vi "initBufferRead.vi"(8 "error in (no error)":errorcluster, 10 "bufferSize":u32=50000, 11 "Electrometer in":refnum<class "Electrometer.lvclass">) -> (0 "error out":errorcluster, 3 "Electrometer out":refnum<class "Electrometer.lvclass">)   [LabVIEW 2016, in "Electrometer.lvclass"]
uses:
  Electrometer.lvclass
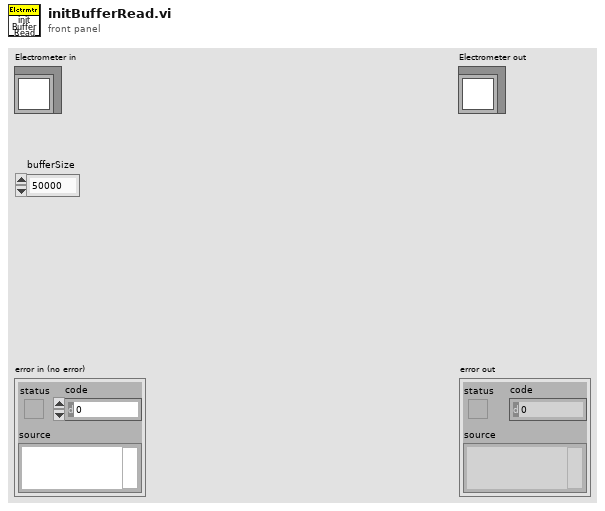
[diagram p1: front panel]
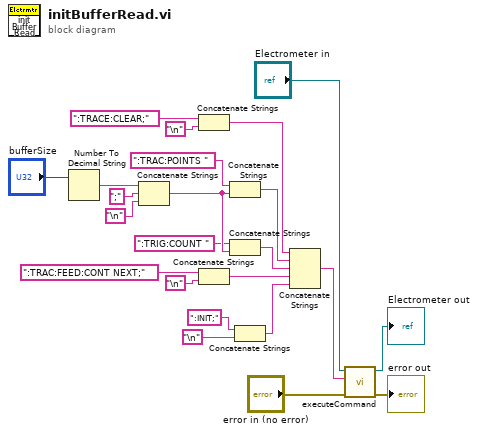
[diagram p0: block diagram]
diagram:
  n1 = Number To Decimal String(number="bufferSize") -> (decimal integer string=w17:string)  [unwired: 1 in]
  n2 = Concatenate Strings(w17, ";" ("string"), "\n") -> (w15:string)
  n3 = Concatenate Strings(":TRACE:CLEAR;" ("command"), "\n") -> (w8:string)
  n4 = Concatenate Strings(":TRAC:FEED:CONT NEXT;" ("command"), "\n") -> (w1:string)
  n5 = Concatenate Strings(":TRAC:POINTS " ("command"), w15) -> (w14:string)
  n6 = Concatenate Strings(":TRIG:COUNT " ("command"), w15) -> (w13:string)
  n7 = Concatenate Strings(":INIT;" ("command"), "\n") -> (w4:string)
  n8 = Concatenate Strings(w8, w14, w13, w1, w4) -> (w12:string)
  n9 = call "executeCommand.vi"("error in (no error)"="error in (no error)", "command"=w12, "Electrometer in"="Electrometer in") -> ("error out"=→"error out":errorcluster, "Electrometer out"=→"Electrometer out":refnum<class "Electrometer.lvclass">)  [unwired: 7 in]
